vi "GV N total pixel clock.vi"() -> ()   [LabVIEW 2017]
panel:
  out "N total pixel clock":u16
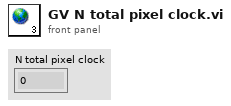
[diagram p1: front panel]
diagram:
